vi "niRFUtil RFHS Apply LUT DPD.vi"(0 "Waveform In (V)":T1 {"y" format="%.2f"; "dx" format="%^.2e"; "x0" format="%^.2e"}, 1 "LUT:LUT Type":enum16{"Log", "Linear"}(ring), 5 "LUT DPD Factor":T2 format="%.2f", 7 "LUT Min Power (dBm)":sgl=-40.0, 9 "LUT Step Size (dB)":sgl=0.1, 11 "error in (no error)":errorcluster) -> (4 "Waveform Out (V)":T1 {"y" format="%.2f"; "dx" format="%^.2e"; "x0" format="%^.2e"}, 15 "error out":errorcluster)   [LabVIEW 2015, in "niRFUtil.lvlib"]
uses:
  niRFUtil.lvlib
  Includes/niRFUtil INC Complex Array.ctl
  Includes/niRFUtil INC Complex Waveform.ctl
  Conversion/niRFUtil CONV 1 Ohm Voltage to 1 Ohm Watt (complex array).vi
panel:
  out "AVX":csg[](array[numeric])
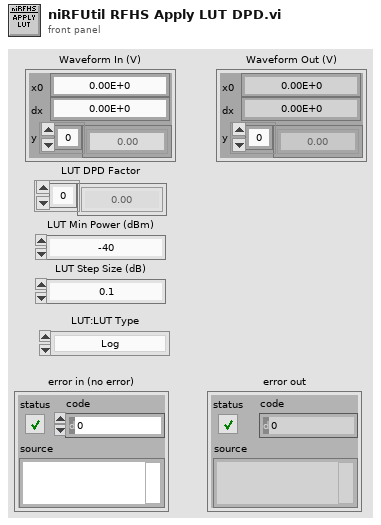
[diagram p1: front panel]
types:
  T1 = typedef "niRFUtil.lvlib/niRFUtil INC Complex Waveform.ctl" = cluster{"x0":dbl, "dx":dbl, "y":T2}
  T2 = typedef "niRFUtil.lvlib/niRFUtil INC Complex Array.ctl" = csg[]
  T3 = typedef "niRFUtil.lvlib/niRFUtil INC Real Array.ctl" = sgl[]
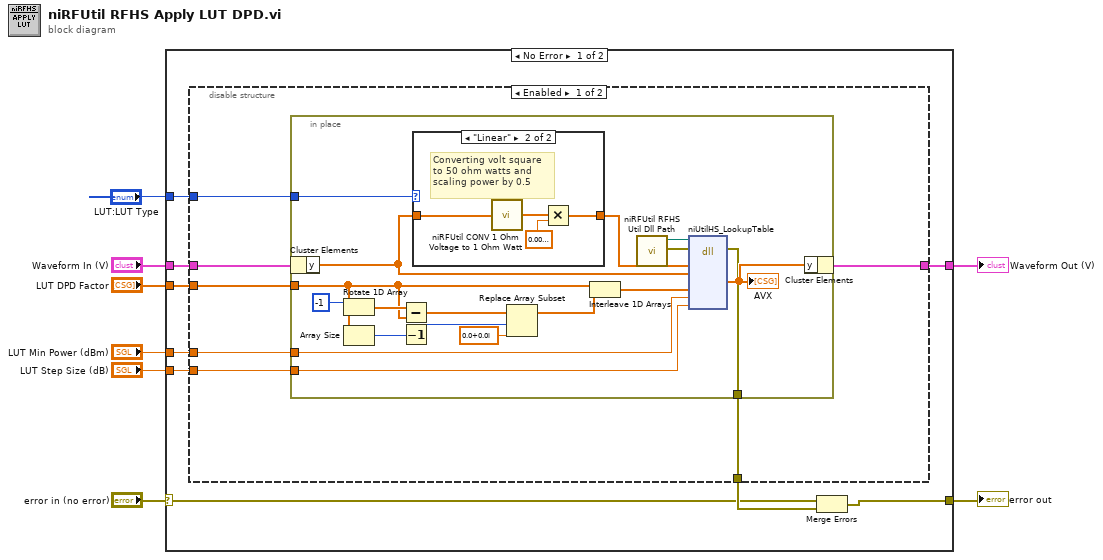
[diagram p0: block diagram]
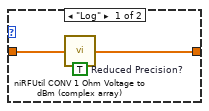
[diagram p2: hidden frame]
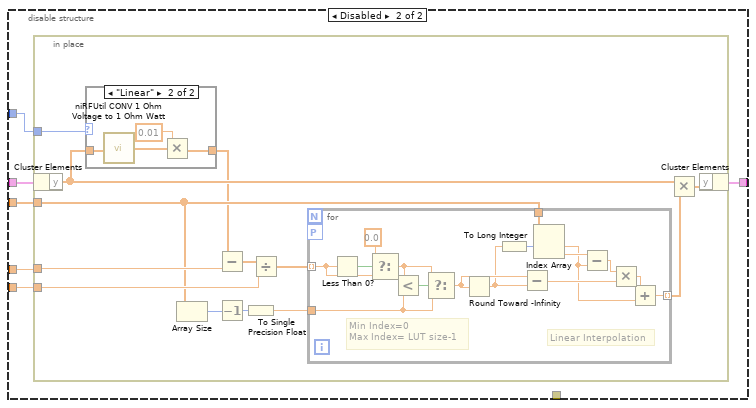
[diagram p3: hidden frame]
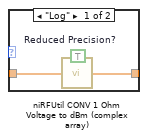
[diagram p4: hidden frame]
diagram:
  n1 = case shown="No Error" "error in (no error)" {
    selector: "error in (no error)" -> [w10 w93]
    tunnel: "LUT Min Power (dBm)" -> [w17 _]
    tunnel: "LUT Step Size (dB)" -> [w16 _]
    tunnel: "LUT DPD Factor" -> [w15 _]
    tunnel: "Waveform In (V)" -> [w14 w92]
    tunnel: [w13 w92] -> w4
    tunnel: [w9 w93] -> w2
    tunnel: "LUT:LUT Type" -> [w12 _]
    frame No Error {
      n2 = disable-structure shown="Enabled" {
        disable-tunnel: w17 -> [w24 w53]
        disable-tunnel: w16 -> [w23 w52]
        disable-tunnel: w15 -> [w22 w54]
        disable-tunnel: w14 -> [w21 w55]
        disable-tunnel: [w20 w51] -> w13
        disable-tunnel: w12 -> [w19 w50]
        disable-tunnel: [w18 _] -> w11
        frame Enabled {
          n3 = in-place {
            in-place-border: w24 -> [w27]
            in-place-border: w23 -> [w42]
            in-place-border: w22 -> [w33]
            in-place-border: w19 -> [w26]
            in-place-border: [w25] -> w18
            n4 = in-place-cluster #1(w21) -> ("y"=w30:T2)
            n5 = Rotate 1D Array(1:w33, 2:-1 ("n")) -> (0:w40:T2)
            n6 = Array Size(array=w33) -> (size(s)=w37:i32)
            n7 = Subtract(x=w40, y=w33) -> (x-y=w39:T2)
            n8 = Decrement(x=w37) -> (x-1=w38:i32)
            n9 = case shown="\"Linear\"" w26 {
              tunnel: w30 -> [w45 w49]
              tunnel: [w44 w46] -> w29
              frame "Log" {
                w43 = TRUE  # Reduced Precision?
                n10 = call "niRFUtil CONV 1 Ohm Voltage to dBm (complex array).vi"("Reduced Precision?"=w43, "Complex Array (V)"=w45) -> ("Real Array (dBm)"=w44:T3)  [unwired: 13 in]
              }
              frame "Linear" {
                # "Converting volt square\nto 50 ohm watts and \nscaling power by 0.5"
                n11 = call-poly "niRFUtil CONV 1 Ohm Voltage to 1 Ohm Watt.vi"("Complex Array (V)"=w49) -> ("Real Array (W)"=w47:T3)  [unwired: 14 in]
                n12 = Multiply(x=w47, y=sgl 0.01) -> (x*y=w46:T3)
              }
            }
            n13 = Replace Array Subset(array=w39, new element=csg 0.0+0.0i ("new element/subarray"), index=w38) -> (w35:T2)
            n14 = Interleave 1D Arrays(w33, w35) -> (w34:T2)
            n15 = call "niRFUtil RFHS Util Dll Path.vi"() -> ("error out"=w31:errorcluster, "Path"=w32:path)  [unwired: 7 in, 3 out]
            n16 = dll-call lib="niRFHS_avx.*" fn="niUtilHS_LookupTable"(path in=w32, error in=w31, "iBuf"=w29, "iWav"=w30, "LUTData"=w34, "a"=w27, "b"=w42) -> (error out=w25:errorcluster, "AVX"=w28:csg[])  [unwired: 8 in, 1 out]
            "AVX" <- w28
            n17 = in-place-cluster #1("y"=w28) -> (w20:T1)
          }
        }
        frame Disabled {
          n18 = in-place {
            in-place-border: w53 -> [w67]
            in-place-border: w52 -> [w66]
            in-place-border: w54 -> [w60]
            in-place-border: w50 -> [w57]
            n19 = in-place-cluster #2(w55) -> ("y"=w58:T2)
            n20 = case shown="\"Linear\"" w57 {
              tunnel: w58 -> [w71 w75]
              tunnel: [w70 w72] -> w56
              frame "Log" {
                w69 = TRUE  # Reduced Precision?
                n21 = call "niRFUtil CONV 1 Ohm Voltage to dBm (complex array).vi"("Reduced Precision?"=w69, "Complex Array (V)"=w71) -> ("Real Array (dBm)"=w70:T3)  [unwired: 13 in]
              }
              frame "Linear" {
                n22 = call-poly "niRFUtil CONV 1 Ohm Voltage to 1 Ohm Watt.vi"("Complex Array (V)"=w75) -> ("Real Array (W)"=w73:T3)  [unwired: 14 in]
                n23 = Multiply(x=0.01, y=w73) -> (x*y=w72:dbl[])
              }
            }
            n24 = Array Size(array=w60) -> (size(s)=w59:i32)
            n25 = Subtract(x=w56, y=w67) -> (x-y=w68:dbl[])
            n26 = Decrement(x=w59) -> (x-1=w62:i32)
            n27 = To Single Precision Float(number=w62) -> (single precision float=w61:sgl)
            n28 = Divide(x=w68, y=w66) -> (x/y=w65:dbl[])
            n29 = for {
              tunnel: w60 -> [w86]
              tunnel: [w85] -> w64 mode=indexing
              tunnel: w65 -> [w80] mode=indexing
              tunnel: w61 -> [w83]
              workers-P: _ -> [_]
              # "Linear Interpolation"
              # "Min Index=0\nMax Index= LUT size-1"
              n30 = Less Than 0?(x=w80) -> (x < 0?=w81:bool)
              n31 = Select(t=sgl 0.0, s=w81, f=w80) -> (s? t:f=w78:dbl)
              n32 = Less?(x=w78, y=w83) -> (x < y?=w84:bool)
              n33 = Select(t=w78, s=w84, f=w83) -> (s? t:f=w82:dbl)
              n34 = Round Toward -Infinity(1:w82) -> (0:w76:dbl)
              n35 = To Long Integer(number=w76) -> (32bit integer=w77:i32)
              n36 = Subtract(x=w82, y=w76) -> (x-y=w89:dbl)
              n37 = Index Array(array=w86, index #1=w77) -> (element #1=w87:csg, element #2=w91:csg)  [unwired: 1 in]
              n38 = Subtract(x=w91, y=w87) -> (x-y=w90:csg)
              n39 = Multiply(x=w90, y=w89) -> (x*y=w88:cdb)
              n40 = Add(x=w88, y=w87) -> (x+y=w85:cdb)
            }
            n41 = Multiply(x=w58, y=w64) -> (x*y=w63:cdb[])
            n42 = in-place-cluster #2("y"=w63) -> (w51:T1)
          }
        }
      }
      n43 = Merge Errors(w10, w11) -> (w9:errorcluster)
    }
    frame Error {
    }
  }
  "Waveform Out (V)" <- w4
  "error out" <- w2
